vi "IC_LiveStart.vi"(1 "ICImagingControl 3":refnum<k7>) -> (0 "ICImagingControl 2":refnum<k7>)   [LabVIEW 2020]
doc: "This VI tries to start a live video stream. It checks whether a valid video capture device has been openen and no live stream is currently running. In case one of these conditions are not fullfilled, nothing happens."
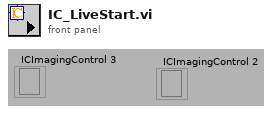
[diagram p1: front panel]
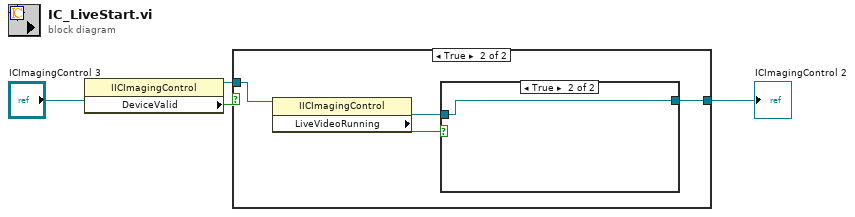
[diagram p0: block diagram]
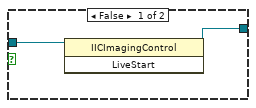
[diagram p3: hidden frame]
diagram:
  n1 = property class="IICImagingControl"(reference="ICImagingControl 3") -> (reference out=w4:refnum<k7>, "DeviceValid"=w3:bool)  [unwired: 1 in, 1 out]
  n2 = case shown="True" w3 {
    tunnel: w4 -> [w5 w9]
    tunnel: [w5 w6] -> w1
    frame False {
    }
    frame True {
      n3 = property class="IICImagingControl"(reference=w9) -> (reference out=w7:refnum<k7>, "LiveVideoRunning"=w8:bool)  [unwired: 1 in, 1 out]
      n4 = case shown="True" w8 {
        tunnel: w7 -> [w11 w12]
        tunnel: [w10 w12] -> w6
        frame False {
          n5 = invoke class="IICImagingControl" method="LiveStart"(reference=w11) -> (reference out=w10:refnum<k7>)  [unwired: 2 in, 2 out]
        }
        frame True {
        }
      }
    }
  }
  "ICImagingControl 2" <- w1
